vi "PNS relevante VIs neu laden.vi"(8 "Fehler (Eingang, kein Fehler)":errorcluster) -> (0 "Fehler (Ausgang)":errorcluster)   [LabVIEW 2020, in "PNS.lvlib" / "Komm Modbus.lvlib"]
uses:
  Komm Modbus.lvlib
  Bildwechsel/Bild-Auswahl.ctl
  VI Anlagengrenzwerte PNS.vi
  PNS.lvlib
  Bildwechsel/Bildwechsel.lvlib
  Allgemein/allgemeine Sub-VIs.lvlib
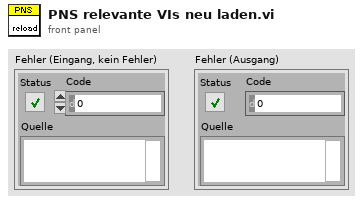
[diagram p1: front panel]
types:
  T1 = enum32{"Bad", "Idle", "Run top level", "Running"}
  T2 = typedef "Bildwechsel.lvlib/Bild-Auswahl.ctl" = enum16{"lesen", "Initialisieren", "Beenden", "Grafik", "Anlagenübersicht", "Anlagengrenzwerte", "Log Konfig", "Gaszuordnung AO", "Erw. Konfiguration", "FT-IR  ", "Störmeldungen", "Störmeldepuffer", "Störmeldekonfig", "PNS Grenzwerte", "Statusübersicht", "Linearisierung", "ARN", "EPA Dichtheitstest", "FID", "PMA", "CalGas", "Lambda", "Interference", "Amium PNS"}
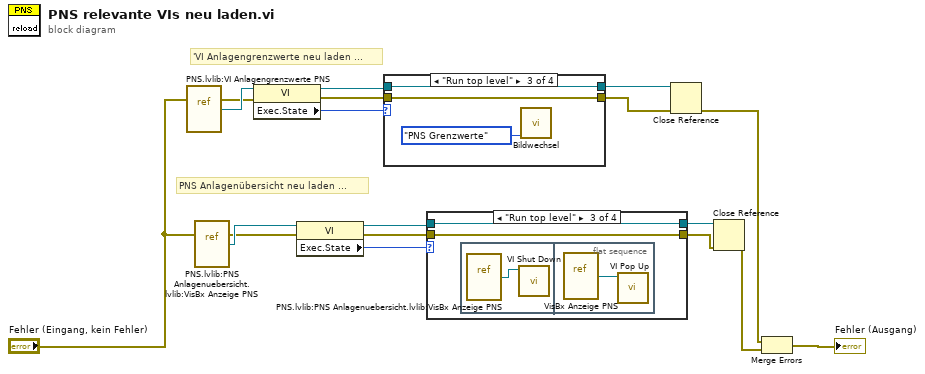
[diagram p0: block diagram]
diagram:
  # "PNS Anlagenübersicht neu laden ..."
  # "'VI Anlagengrenzwerte neu laden ..."
  n1 = vi-ref "PNS.lvlib:VI Anlagengrenzwerte PNS.vi"() -> (w11:refnum<vi>)
  n2 = vi-ref "PNS.lvlib:PNS Anlagenuebersicht.lvlib:VisBx Anzeige PNS.vi"() -> (w4:refnum<vi>)
  n3 = property class="VI"(reference=w11, error in="Fehler (Eingang, kein Fehler)") -> (reference out=w13:refnum<vi>, error out=w14:errorcluster, "Exec.State"=w12:T1)
  n4 = property class="VI"(reference=w4, error in="Fehler (Eingang, kein Fehler)") -> (reference out=w7:refnum<vi>, error out=w8:errorcluster, "Exec.State"=w6:T1)
  n5 = case shown="\"Run top level\"" w12 {
    tunnel: w13 -> [w17 w19 w22 w24]
    tunnel: w14 -> [w18 w20 w21 w25]
    tunnel: [w17 w19 w22 w24] -> w15
    tunnel: [w18 w20 w21 w25] -> w16
    frame "Bad", Default {
    }
    frame "Idle" {
    }
    frame "Run top level" {
      n6 = call "Bildwechsel.vi"("nächstes Bild"=Bild-Auswahl."PNS Grenzwerte") -> ()  [unwired: 9 in, 2 out]
    }
    frame "Running" {
    }
  }
  n7 = case shown="\"Run top level\"" w6 {
    tunnel: w7 -> [w26 w28 w31 w34]
    tunnel: w8 -> [w27 w29 w30 w35]
    tunnel: [w26 w28 w31 w34] -> w9
    tunnel: [w27 w29 w30 w35] -> w10
    frame "Bad", Default {
    }
    frame "Idle" {
    }
    frame "Run top level" {
      n8 = flat-sequence {
        frame #0 {
          n9 = vi-ref "PNS.lvlib:PNS Anlagenuebersicht.lvlib:VisBx Anzeige PNS.vi"() -> (w32:refnum<vi>)
          n10 = call "VI Shut Down.vi"("VI Referenz"=w32) -> ()  [unwired: 11 in]
        }
        frame #1 {
          n11 = vi-ref "VisBx Anzeige PNS.vi"() -> (w33:refnum<vi>)
          n12 = call "VI Pop Up.vi"("VI Referenz"=w33) -> ()  [unwired: 11 in]
        }
      }
    }
    frame "Running" {
    }
  }
  n13 = Close Reference(reference=w15, error in (no error)=w16) -> (error out=w1:errorcluster)
  n14 = Close Reference(reference=w9, error in (no error)=w10) -> (error out=w5:errorcluster)
  n15 = Merge Errors(w1, w5) -> (→"Fehler (Ausgang)":errorcluster)
